vi "Demo.vi"   [LabVIEW 2021]
doc: "本VI是为《我和LabVIEW》一书编写的示例。\n关于本书的介绍请参考网页：\nhttp://ruanqizhen.spaces.live.com/blog/cns!5852D4F797C53FB6!4310.entry"
uses:
  PluginInterface/PluginInterface.lvclass
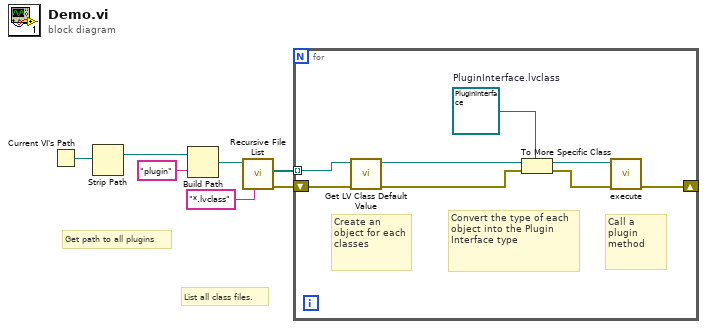
[diagram p0: block diagram]
diagram:
  # "List all class files."
  # "Get path to all plugins"
  n1 = Current VI's Path() -> (path=w7:path)
  n2 = Strip Path(path=w7) -> (stripped path=w6:path)  [unwired: 1 out]
  n3 = Build Path(base path=w6, name or relative path="plugin" ("名称或相对路径")) -> (appended path=w4:path)
  n4 = call <vilib>:"Recursive File List.vi"("pattern"="*.lvclass" ("模式"), "Folder Path"=w4) -> ("error out"=w1:errorcluster, "All Files in Dir"=w3:path[])  [unwired: 2 in, 6 out]
  n5 = for {
    tunnel: w3 -> [w15] mode=indexing
    shift-right: [w8] -> _
    shift-left: w1 -> [w12]
    w11 = refnum<class "PluginInterface.lvclass"> refnum  # PluginInterface.lvclass
    # "Call a plugin method"
    # "Convert the type of each object into the Plugin Interface type"
    # "Create an object for each classes"
    n6 = call <vilib>:"Get LV Class Default Value.vi"("error in (no error)"=w12, "class path"=w15) -> ("error out"=w13:errorcluster, "object"=w14:refnum<class>)  [unwired: 8 out]
    n7 = To More Specific Class(target class=w11, reference=w14, error in=w13) -> (specific class reference=w10:refnum<class "PluginInterface.lvclass">, error out=w9:errorcluster)
    n8 = call-dynamic "execute.vi"("error in (no error)"=w9, "PluginInterface.lvclass"=w10) -> ("error out"=w8:errorcluster)  [unwired: 8 in, 1 out]
  }
